vi "Uniform (Discrete) Random.vi"(6 "seed":i32=-1, 7 "reset":bool, 10 "n":i32=100, 11 "samples":i32=128) -> (0 "error":i32, 3 "uniform (discrete) random data":i32[](array[numeric]))   [LabVIEW 2020, in "NI_Gmath.lvlib"]
doc: "Generates random values from a variate X, where X describes the selected distribution type. You must manually select the polymorphic instance to use."
uses:
  <vilib>/gmath/NI_Gmath.lvlib
panel:
  # "Uniform (Discrete) Random"
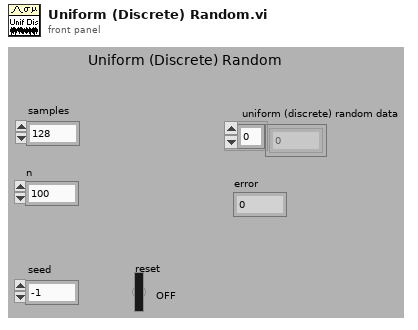
[diagram p1: front panel]
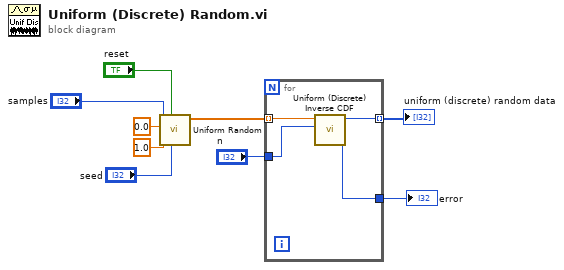
[diagram p0: block diagram]
diagram:
  n1 = call <vilib>:"Uniform Random.vi"("seed"="seed", "reset"="reset", "xmax"=1.0, "xmin"=0.0, "samples"="samples") -> ("uniform random data"=w3:dbl[])  [unwired: 5 in, 1 out]
  n2 = for {
    tunnel: w3 -> [w13] mode=indexing
    tunnel: "n" -> [w10]
    tunnel: [w12] -> w8 mode=indexing
    tunnel: [w11] -> w7
    n3 = call <vilib>:"Uniform (Discrete) Inverse CDF.vi"("n"=w10, "cdf(x)"=w13) -> ("error"=w11:i32, "x"=w12:i32)  [unwired: 8 in]
  }
  "error" <- w7
  "uniform (discrete) random data" <- w8
